vi "MVC Collection Finished.vi"(8 "error in (no error)":errorcluster, 10 "Cluster":cluster{"Left":dbl, "Right":dbl} {"Right" format="%#_13g"; "Left" format="%#_13g"}, 11 "GUI in":refnum<class "GUI.lvclass">) -> (0 "error out":errorcluster, 3 "GUI out":refnum<class "GUI.lvclass">)   [LabVIEW 2020, in "GUI.lvlib" / "GUI.lvclass"]
uses:
  GUI.lvclass
  GUI.lvclass/GUI.ctl
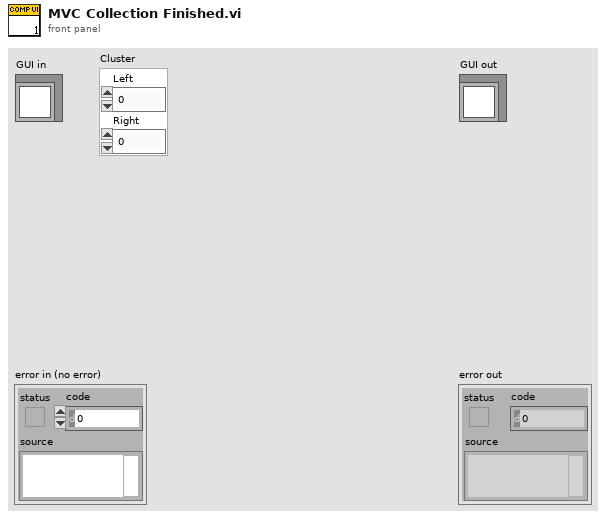
[diagram p1: front panel]
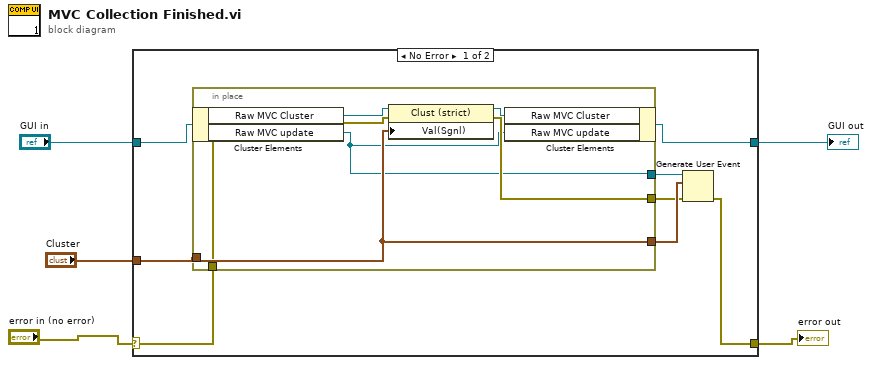
[diagram p0: block diagram]
diagram:
  n1 = case shown="No Error" "error in (no error)" {
    selector: "error in (no error)" -> [w8 w20]
    tunnel: [w6 w21] -> w4
    tunnel: "GUI in" -> [w13 w21]
    tunnel: [w7 w20] -> w2
    tunnel: "Cluster" -> [w12 _]
    frame No Error {
      n2 = in-place {
        in-place-border: w12 -> [w17]
        in-place-border: [w14] -> w11
        in-place-border: [w17] -> w10
        in-place-border: [w16] -> w9
        in-place-border: w8 -> [w15]
        n3 = in-place-cluster #1(w13) -> ("Raw MVC Cluster"=w19:refnum<vi>, "Raw MVC update"=w14:refnum<user-event>)
        n4 = property class="Clust (strict)"(reference=w19, error in=w15, "Val(Sgnl)"=w17) -> (reference out=w18:refnum<vi>, error out=w16:errorcluster)
        n5 = in-place-cluster #1("Raw MVC Cluster"=w18, "Raw MVC update"=w14) -> (w6:refnum<class "GUI.lvclass">)
      }
      n6 = Generate User Event(user event=w11, event data cluster=w10, error in=w9) -> (error out=w7:errorcluster)  [unwired: 1 in, 1 out]
    }
    frame Error {
    }
  }
  "error out" <- w2
  "GUI out" <- w4
